vi "RWA_String Section To Anything.vi"(5 "Format String (%#_13g)":string="%#_13g", 6 "Use Supplied":bool, 7 "Read/Write Options":T1={"TS Fmt"="", "Int Fmt"="", "Delimiter"=","}, 8 "Error":errorcluster, 9 "String Section":string, 11 "Type Of Anything":variant) -> (0 "Error Out":errorcluster, 2 "Read Failures Out":string, 3 "Type Of Anything Out":variant, 4 "All Items Found Out":bool)   [LabVIEW 2020]
doc: "Parse the specified String to populate the specified datatype. If string doesn't contain a field defined by datatype, then that field is set based on \"Use Supplied\". If \"Use Supplied\" is true, then the field is left as is, otherwise the field is set to default value.\n\nAuthored by Robert C. Mortensen\nsupport@mooregoodideas.com\nwww.mooregoodideas.com\n\nCopyright (c) 2010, Moore Good Ideas, Inc.\n\nAll rights reserved.\n\nRedistribution and use in source and binary forms, with or without modification, are permitted provided that the following conditions are met:\n\n * Redistributions of source code must retain the above copyright notice, this list of conditions and the following disclaimer.\n * Redistributions in binary form must reproduce the above copyright notice, this list of conditions and the following disclaimer in the documentation and/or other materials provided with the distribution.\n * Neither the name of Moore Good Ideas, Inc. nor the names of its contributors may be used to endorse or promote products derived from this software without specific prior written permission.\n\nTHIS SOFTWARE IS PROVIDED BY THE COPYRIGHT HOLDERS AND CONTRIBUTORS \"AS IS\" AND ANY EXPRESS OR IMPLIED WARRANTIES, INCLUDING, BUT NOT LIMITED TO, THE IMPLIED WARRANTIES OF MERCHANTABILITY AND FITNESS FOR A PARTICULAR PURPOSE ARE DISCLAIMED. IN NO EVENT SHALL THE COPYRIGHT OWNER OR CONTRIBUTORS BE LIABLE FOR ANY DIRECT, INDIRECT, INCIDENTAL, SPECIAL, EXEMPLARY, OR CONSEQUENTIAL DAMAGES (INCLUDING, BUT NOT LIMITED TO, PROCUREMENT OF SUBSTITUTE GOODS OR SERVICES; LOSS OF USE, DATA, OR PROFITS; OR BUSINESS INTERRUPTION) HOWEVER CAUSED AND ON ANY THEORY OF LIABILITY, WHETHER IN CONTRACT, STRICT LIABILITY, OR TORT (INCLUDING NEGLIGENCE OR OTHERWISE) ARISING IN ANY WAY OUT OF THE USE OF THIS SOFTWARE, EVEN IF ADVISED OF THE POSSIBILITY OF SUCH DAMAGE."
uses:
  MGI RWA Options Cluster.ctl
  MGI RWA Convertion Direction Enum.ctl
  <vilib>/Utility/VariantDataType/Type.ctl
  String/MGI Scan From String/MGI Scan From String (CDB).vi
  String/MGI Scan From String/MGI Scan From String (CSG).vi
  String/MGI Scan From String/MGI Scan From String (CXT).vi
  <vilib>/Utility/VariantDataType/VariantType.lvlib
  <vilib>/Utility/Data Type/NI_Data Type.lvlib
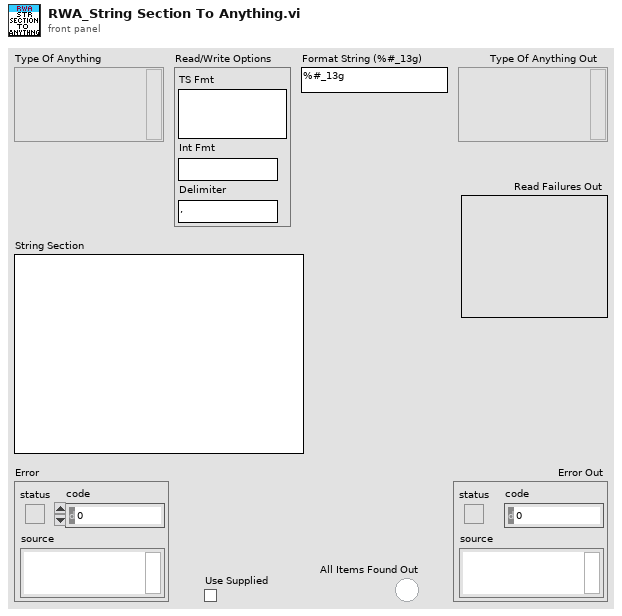
[diagram p1: front panel]
types:
  T1 = typedef "MGI RWA Options Cluster.ctl" = cluster{"TS Fmt":string, "Int Fmt":string, "Delimiter":string}
  T2 = typedef "MGI RWA Convertion Direction Enum.ctl" = enum16{"String->Anything", "Anything->String"}
  T3 = typedef "MGI RWA Tag Lookup Cluster.ctl" = cluster{"StrToSpecifiedText":variant, "Specified Data":variant, "Float Fmt":string, "Major Vers":i32, "Options":T1}
  T4 = typedef "VariantType.lvlib/Type.ctl" = enum8{"Invalid Type", "Void", "I8", "I16", "I32", "I64", "U8", "U16", "U32", "U64", "Single Float", "Double Float", "Extended Float", "Single Complex", "Double Complex", "Extended Complex", "Enum U8", "Enum U16", "Enum U32", "Enum U64", "Single Float With Unit", "Double Float With Unit", "Extended Float With Unit", "Single Complex with Unit", "Double Complex with Unit", "Extended Complex with Unit", "Boolean", "String", "Path", "Picture", "Tag", "Array", "Cluster", "Variant", "LV Variant", "Waveform", "Timestamp", "Digital Waveform", "Digital Data", "ExpressData", "Refnum", "External Data", "VI", "Poly VI", "LabVIEW Class Instance", "Fixed Point"}
  T5 = typedef "NI_Data Type.lvlib/Data Type.ctl" = enum8{"Invalid Type", "Void", "I8", "I16", "I32", "I64", "U8", "U16", "U32", "U64", "Single Float", "Double Float", "Extended Float", "Single Complex", "Double Complex", "Extended Complex", "Enum U8", "Enum U16", "Enum U32", "Enum U64", "Single Float With Unit", "Double Float With Unit", "Extended Float With Unit", "Single Complex with Unit", "Double Complex with Unit", "Extended Complex with Unit", "Boolean", "String", "Path", "Picture", "Tag", "Array", "Cluster", "Variant", "LV Variant", "Waveform", "Timestamp", "Digital Waveform", "Digital Data", "ExpressData", "Refnum", "External Data", "VI", "Poly VI", "LabVIEW Class Instance", "Fixed Point", "Set Collection", "Map Collection"}
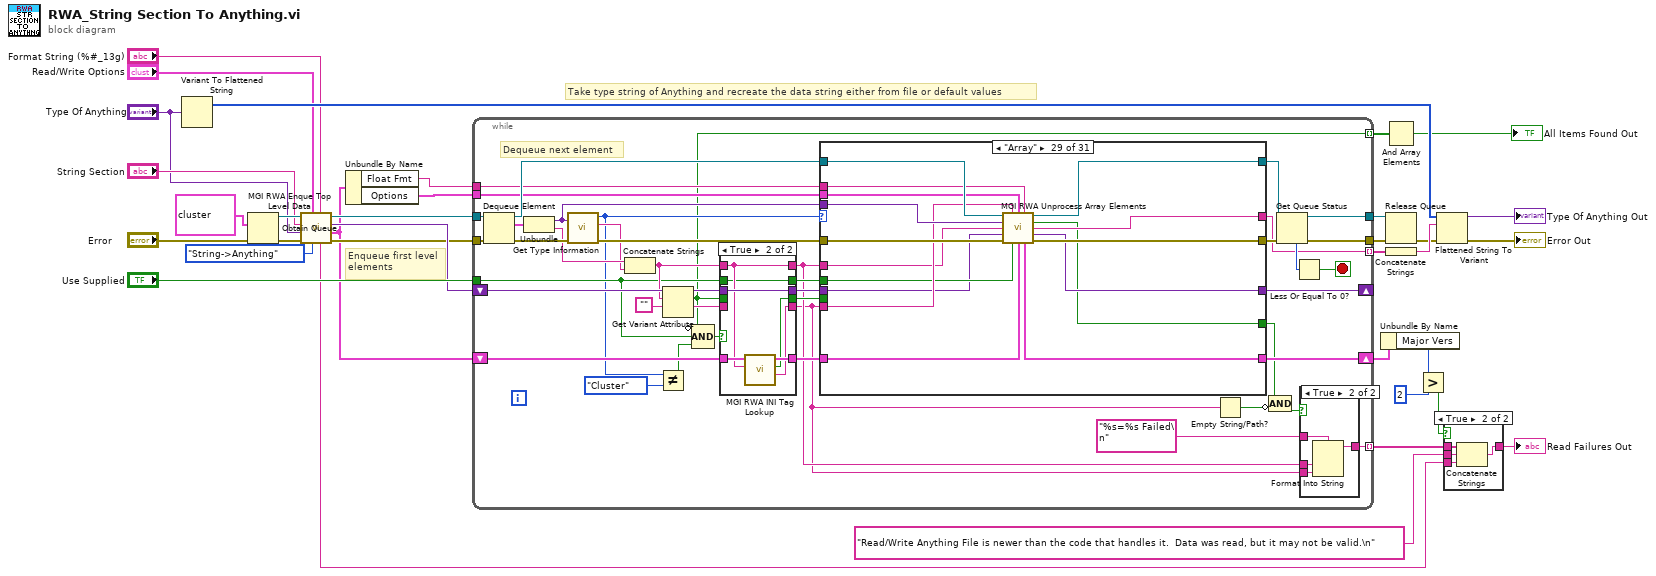
[diagram p0: block diagram]
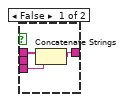
[diagram p2: hidden frame]
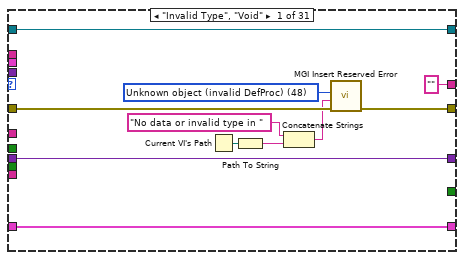
[diagram p5: hidden frame]
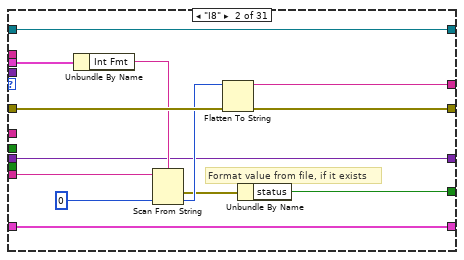
[diagram p6: hidden frame]
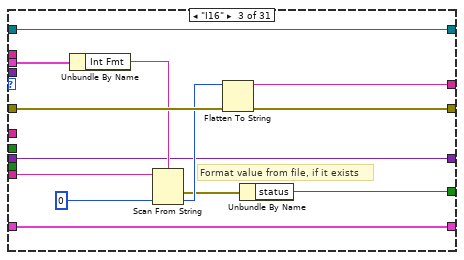
[diagram p7: hidden frame]
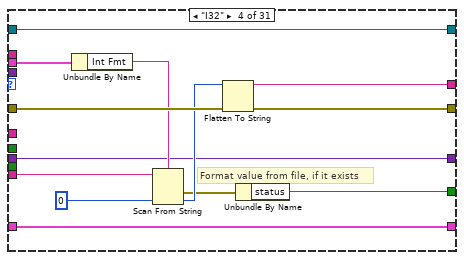
[diagram p8: hidden frame]
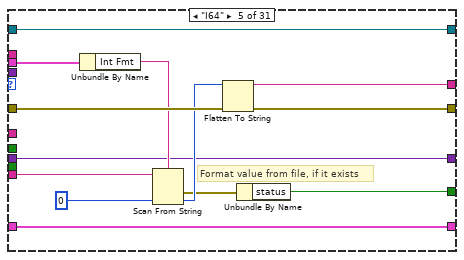
[diagram p9: hidden frame]
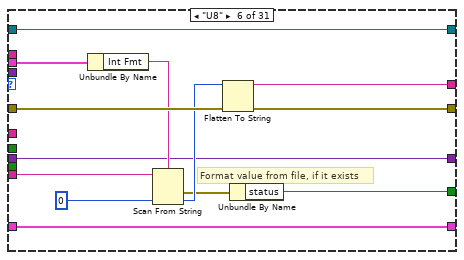
[diagram p10: hidden frame]
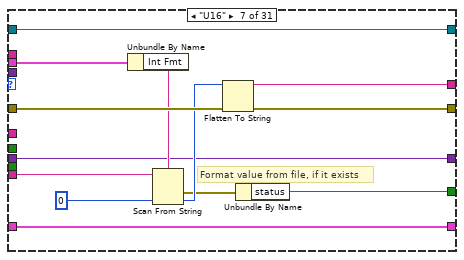
[diagram p11: hidden frame]
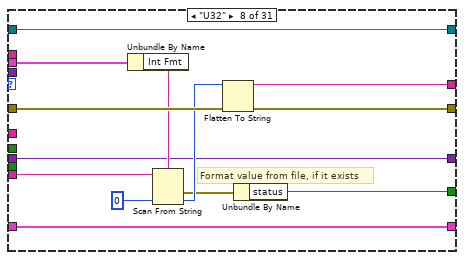
[diagram p12: hidden frame]
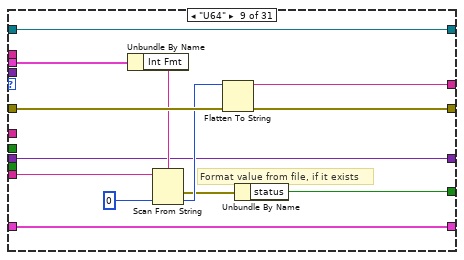
[diagram p13: hidden frame]
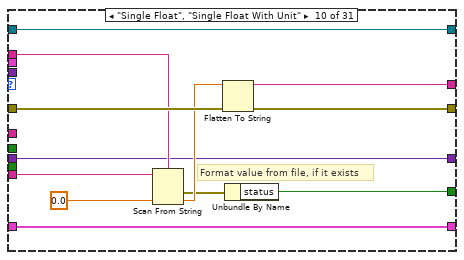
[diagram p14: hidden frame]
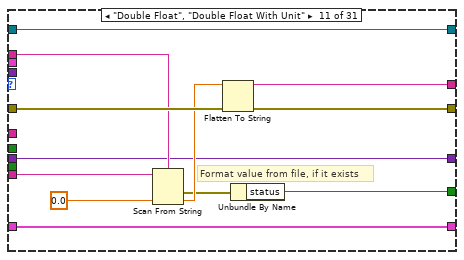
[diagram p15: hidden frame]
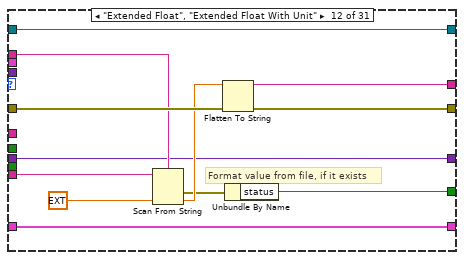
[diagram p16: hidden frame]
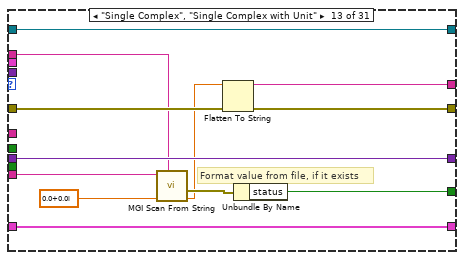
[diagram p17: hidden frame]
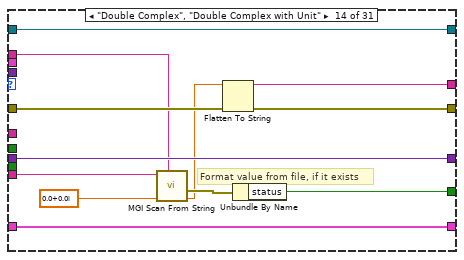
[diagram p18: hidden frame]
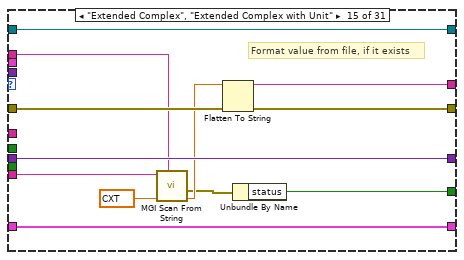
[diagram p19: hidden frame]
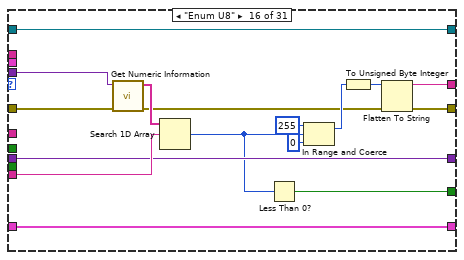
[diagram p20: hidden frame]
diagram:
  # "Enqueue first level\nelements"
  # "Take type string of Anything and recreate the data string either from file or default values"
  n1 = Variant To Flattened String(Variant="Type Of Anything") -> (1:w27:i16[])  [unwired: 1 out]
  n2 = Obtain Queue(element data type=cluster{"Variant":variant, "Name":string} {"Variant"=variant, "Name"=""}, error in (no error)="Error") -> (queue out=w25:refnum<queue>, error out=w19:errorcluster)  [unwired: 3 in, 1 out]
  n3 = call "MGI RWA Enque Top Level Data.vi"("Format String (%#_13g)"="Format String (%#_13g)", "Conversion"=MGI_RWA_Convertion_Direction_Enum."String->Anything", "Read/Write Options"="Read/Write Options", "Error In"=w19, "Anything"="Type Of Anything", "Read String"="String Section", "Data Queue In"=w25) -> ("Error Out"=w22:errorcluster, "Read State"=w17:T3, "Tag to String"=w24:variant, "Data Queue Our"=w23:refnum<queue>, "Warnings"=w3:string)
  n4 = Unbundle By Name(w17) -> ("Float Fmt"=w15:string, "Options"=w13:T1)
  n5 = while {
    tunnel: w22 -> [w76]
    tunnel: [w43] -> w30
    tunnel: [w63] -> w29 mode=indexing
    tunnel: w23 -> [w73]
    tunnel: [w68] -> w32
    tunnel: w13 -> [w45]
    tunnel: w15 -> [w44]
    shift-right: [w50] -> w12
    shift-left: w17 -> [w54]
    shift-right: [w49] -> _
    shift-left: w24 -> [w61]
    tunnel: "Use Supplied" -> [w53]
    tunnel: [w36] -> w8 mode=indexing
    tunnel: [w35] -> w2 mode=indexing
    stop <- w69 stop-if-true
    # "Dequeue next element"
    n6 = Dequeue Element(queue=w73, error in (no error)=w76) -> (queue out=w74:refnum<queue>, element=w67:cluster{"Variant":variant, "Name":string}, error out=w75:errorcluster)  [unwired: 1 in, 1 out]
    n7 = Unbundle(w67) -> ("Variant"=w65:variant, "Name"=w66:string)
    n8 = call <vilib>:"Get Type Information.vi"("error in (no error)"=w75, "variant"=w65) -> ("error out"=w77:errorcluster, "name"=w64:string, "type"=w48:T5)  [unwired: 5 in, 2 out]
    n9 = Concatenate Strings(w66, w64) -> (w58:string)
    n10 = Not Equal?(x=w48, y=Type."Cluster") -> (x != y?=w47:bool)
    n11 = Get Variant Attribute(Variant=w61, name=w58, default value (empty Variant)="") -> (duplicate Variant=w57:variant, found=w35:bool, value=w60:string)  [unwired: 1 in, 1 out]
    n12 = Compound Arithmetic op=AND(invert w35, w53, w47) -> (w59:bool)
    n13 = case shown="True" w59 {
      tunnel: w60 -> [w84 _]
      tunnel: w35 -> [w85 _]
      tunnel: w58 -> [w86 w89]
      tunnel: w57 -> [w87 w93]
      tunnel: [w87 w93] -> w56
      tunnel: [w86 w89] -> w39
      tunnel: [w85 w91] -> w55
      tunnel: [w84 w90] -> w38
      tunnel: w54 -> [w83 w94]
      tunnel: [w83 w92] -> w51
      tunnel: w53 -> [w82 w88]
      tunnel: [w82 w88] -> w52
      frame False {
      }
      frame True {
        n14 = call "MGI RWA INI Tag Lookup.vi"("String"=w89, "State In"=w94) -> ("INI Text"=w90:string, "Text Found?"=w91:bool, "State Out"=w92:T3)  [unwired: 7 in]
      }
    }
    n15 = case shown="\"Array\"" w48 {
      tunnel: [w99 w118 w131 w144 w157 w170 w183 w196 w209 w221 w233 w245 w257 w269 w281 w297 w313 w329 w345 w355 w363 w371 w379 w400 w428 w461 w507 w535 w567 w582 w603] -> w72
      tunnel: w77 -> [w100 w117 w130 w143 w156 w169 w182 w195 w208 w220 w232 w244 w256 w268 w280 w296 w312 w328 w344 w354 w362 w370 w385 w399 w427 w460 w506 w534 w570 w581 w602]
      tunnel: w39 -> [_ _ _ _ _ _ _ _ _ _ _ _ _ _ _ _ _ _ _ _ _ _ w372 _ _ _ _ _ w564 _ _]
      tunnel: ["" ("data string") w116 w129 w142 w155 w168 w181 w194 w207 w219 w231 w243 w255 w267 w279 w295 w311 w327 w343 w353 w361 w369 "" w398 w426 w459 w505 w533 w559 w580 w601] -> w63
      tunnel: w65 -> [_ _ _ _ _ _ _ _ _ _ _ _ _ _ _ w294 w310 w326 w342 _ _ _ w384 _ _ _ _ _ w569 w573 _]
      tunnel: w74 -> [w101 w115 w128 w141 w154 w167 w180 w193 w206 w218 w230 w242 w254 w266 w278 w293 w309 w325 w341 w352 w360 w368 w380 w397 w425 w458 w504 w532 w571 w579 w600]
      tunnel: [w101 w115 w128 w141 w154 w167 w180 w193 w206 w218 w230 w242 w254 w266 w278 w293 w309 w325 w341 w352 w360 w368 w378 w397 w425 w458 w504 w532 w566 w579 w600] -> w71
      tunnel: w56 -> [w96 w110 w123 w136 w149 w162 w175 w188 w202 w213 w225 w237 w253 w265 w277 w285 w301 w318 w333 w347 w358 w365 w374 w395 w422 w451 w501 w529 w563 w574 w597]
      tunnel: w45 -> [_ w108 w121 w134 w147 w160 w173 w186 w199 _ _ _ _ _ _ _ _ _ _ _ _ _ _ _ _ _ _ _ w558 _ _]
      tunnel: w44 -> [_ _ _ _ _ _ _ _ _ w215 w227 w239 w248 w261 w272 _ _ _ _ _ _ _ _ _ _ _ _ _ w557 _ _]
      tunnel: [w96 w110 w123 w136 w149 w162 w175 w188 w202 w213 w225 w237 w253 w265 w277 w285 w301 w318 w333 w347 w358 w365 w374 w395 w422 w451 w501 w529 w560 w574 w597] -> w49
      tunnel: w38 -> [_ w111 w124 w137 w150 w163 w176 w189 w201 w214 w226 w238 w247 w258 w273 w286 w302 w319 w334 w348 w359 w366 _ w396 w424 w452 w502 w530 w568 w577 w598]
      tunnel: w55 -> [_ _ _ _ _ _ _ _ _ _ _ _ _ _ _ _ _ _ _ _ _ _ _ w394 w423 w453 w503 w531 _ w578 w599]
      tunnel: w52 -> [_ _ _ _ _ _ _ _ _ _ _ _ _ _ _ _ _ _ _ _ _ _ _ _ _ _ _ _ w565 _ _]
      tunnel: w51 -> [w95 w109 w122 w135 w148 w161 w174 w187 w200 w212 w224 w236 w252 w264 w276 w284 w300 w317 w332 w346 w357 w364 w373 w393 w421 w450 w500 w528 w562 w576 w596]
      tunnel: [w95 w109 w122 w135 w148 w161 w174 w187 w200 w212 w224 w236 w252 w264 w276 w284 w300 w317 w332 w346 w357 w364 w373 w393 w421 w450 w500 w528 w561 w575 w596] -> w50
      tunnel: [_ w106 w119 w132 w145 w158 w171 w184 w197 w210 w222 w234 w251 w263 w275 w282 w298 w314 w330 _ _ _ _ _ _ w449 _ _ w556 w572 _] -> w42
      frame "Invalid Type", "Void" {
        w97 = u16 48 items=["No error", "Argument error", "Memory is full", "Out of zone", "End of file", "File already open", "Generic file I/O error", "File not found", "File permission error", "Disk is full", "Duplicate path", "Too many files open", "System feature not enabled", "Resource file not found", "Cannot add resource", "Resource not found", "Image not found", "Image memory error", "Pen does not exist", "Config type invalid", "Config token not found", "Config parse error", "Config memory error", "Bad external code format", "Bad external code offset", "External code not present", "Null window", "Destroy window error", "Null menu", "Print aborted", "Bad print record", "Print driver error", "Windows error during printing", "Memory error during printing", "Print dialog error", "Generic print error", "Invalid device refnum", "Device not found", "Device parameter error", "Device unit error", "Cannot open device", "Device call aborted", "Generic error", "Cancelled by user", "Object ID too low", "Object ID too high", "Object not in heap", "Unknown heap", "Unknown object (invalid DefProc)", "Unknown object (DefProc not in table)", "Message out of range", "Invalid (null) method", "Unknown message", "Manager call not supported", "Bad address", "Network operation in progress", "Network operation timed out", "Connection is busy", "Network attribute not supported", "Network error", "Address in use", "System out of memory", "Connection aborted", "Connection refused", "Not connected", "Already connected", "Connection closed", "Initialization error (interapplication manager)", "Bad occurrence", "Wait on unbound occurrence handler", "Occurrence queue overflow", "Datalog type conflict", "Unused", "Unrecognized type (interapplication manager)", "Memory corrupt", "Failed to make temporary DLL", "Old CIN version", "Drag socket not found", "Failed to load drop-object", "Failed to register OLE object", "Failed to release OLE object", "Format specifier type mismatch", "Unknown format specifier", "Too few format specifiers", "Too many format specifiers", "Scan failed", "Newer CIN version", "OLE Convert", "Runtime menu error", "Password tampered", "Unknown error code"] ("Reserved Error Code")
        n16 = Current VI's Path() -> (path=w103:path)
        n17 = Path To String(path=w103) -> (string=w102:string)
        n18 = Concatenate Strings("No data or invalid type in " ("string"), w102) -> (w98:string)
        n19 = call "MGI Insert Reserved Error.vi"("Error In"=w100, "Error Description"=w98, "Reserved Error Code (Generic error)"=w97) -> ("Error Out"=w99:errorcluster)  [unwired: 8 in]
      }
      frame "I8" {
        # "Format value from file, if it exists"
        n20 = Unbundle By Name(w108) -> ("Int Fmt"=w113:string)
        n21 = Scan From String(format string=w113, input string=w111, default 1=i8 0 ("default (0 I32)")) -> (error out=w107:errorcluster, output 1=w112:i8)  [unwired: 2 in, 2 out]
        n22 = Flatten To String(anything=w112, error in (no error)=w117) -> (data string=w116:string, error out=w118:errorcluster)  [unwired: 2 in, 1 out]
        n23 = Unbundle By Name(w107) -> ("status"=w106:bool)
      }
      frame "I16" {
        # "Format value from file, if it exists"
        n24 = Unbundle By Name(w121) -> ("Int Fmt"=w126:string)
        n25 = Scan From String(format string=w126, input string=w124, default 1=i16 0 ("default (0 I32)")) -> (error out=w120:errorcluster, output 1=w125:i16)  [unwired: 2 in, 2 out]
        n26 = Flatten To String(anything=w125, error in (no error)=w130) -> (data string=w129:string, error out=w131:errorcluster)  [unwired: 2 in, 1 out]
        n27 = Unbundle By Name(w120) -> ("status"=w119:bool)
      }
      frame "I32" {
        # "Format value from file, if it exists"
        n28 = Unbundle By Name(w134) -> ("Int Fmt"=w139:string)
        n29 = Scan From String(format string=w139, input string=w137, default 1=0 ("default (0 I32)")) -> (error out=w133:errorcluster, output 1=w138:i32)  [unwired: 2 in, 2 out]
        n30 = Flatten To String(anything=w138, error in (no error)=w143) -> (data string=w142:string, error out=w144:errorcluster)  [unwired: 2 in, 1 out]
        n31 = Unbundle By Name(w133) -> ("status"=w132:bool)
      }
      frame "I64" {
        # "Format value from file, if it exists"
        n32 = Unbundle By Name(w147) -> ("Int Fmt"=w152:string)
        n33 = Scan From String(format string=w152, input string=w150, default 1=i64 0 ("default (0 I32)")) -> (error out=w146:errorcluster, output 1=w151:i64)  [unwired: 2 in, 2 out]
        n34 = Flatten To String(anything=w151, error in (no error)=w156) -> (data string=w155:string, error out=w157:errorcluster)  [unwired: 2 in, 1 out]
        n35 = Unbundle By Name(w146) -> ("status"=w145:bool)
      }
      frame "U8" {
        # "Format value from file, if it exists"
        n36 = Unbundle By Name(w160) -> ("Int Fmt"=w165:string)
        n37 = Scan From String(format string=w165, input string=w163, default 1=u8 0 ("default (0 I32)")) -> (error out=w159:errorcluster, output 1=w164:u8)  [unwired: 2 in, 2 out]
        n38 = Flatten To String(anything=w164, error in (no error)=w169) -> (data string=w168:string, error out=w170:errorcluster)  [unwired: 2 in, 1 out]
        n39 = Unbundle By Name(w159) -> ("status"=w158:bool)
      }
      frame "U16" {
        # "Format value from file, if it exists"
        n40 = Unbundle By Name(w173) -> ("Int Fmt"=w178:string)
        n41 = Scan From String(format string=w178, input string=w176, default 1=u16 0 ("default (0 I32)")) -> (error out=w172:errorcluster, output 1=w177:u16)  [unwired: 2 in, 2 out]
        n42 = Flatten To String(anything=w177, error in (no error)=w182) -> (data string=w181:string, error out=w183:errorcluster)  [unwired: 2 in, 1 out]
        n43 = Unbundle By Name(w172) -> ("status"=w171:bool)
      }
      frame "U32" {
        # "Format value from file, if it exists"
        n44 = Unbundle By Name(w186) -> ("Int Fmt"=w191:string)
        n45 = Scan From String(format string=w191, input string=w189, default 1=u32 0 ("default (0 I32)")) -> (error out=w185:errorcluster, output 1=w190:u32)  [unwired: 2 in, 2 out]
        n46 = Flatten To String(anything=w190, error in (no error)=w195) -> (data string=w194:string, error out=w196:errorcluster)  [unwired: 2 in, 1 out]
        n47 = Unbundle By Name(w185) -> ("status"=w184:bool)
      }
      frame "U64" {
        # "Format value from file, if it exists"
        n48 = Unbundle By Name(w199) -> ("Int Fmt"=w204:string)
        n49 = Scan From String(format string=w204, input string=w201, default 1=u64 0 ("default (0 I32)")) -> (error out=w198:errorcluster, output 1=w203:u64)  [unwired: 2 in, 2 out]
        n50 = Flatten To String(anything=w203, error in (no error)=w208) -> (data string=w207:string, error out=w209:errorcluster)  [unwired: 2 in, 1 out]
        n51 = Unbundle By Name(w198) -> ("status"=w197:bool)
      }
      frame "Single Float", "Single Float With Unit" {
        # "Format value from file, if it exists"
        n52 = Scan From String(format string=w215, input string=w214, default 1=sgl 0.0 ("default (0 I32)")) -> (error out=w211:errorcluster, output 1=w216:sgl)  [unwired: 2 in, 2 out]
        n53 = Flatten To String(anything=w216, error in (no error)=w220) -> (data string=w219:string, error out=w221:errorcluster)  [unwired: 2 in, 1 out]
        n54 = Unbundle By Name(w211) -> ("status"=w210:bool)
      }
      frame "Double Float", "Double Float With Unit" {
        # "Format value from file, if it exists"
        n55 = Scan From String(format string=w227, input string=w226, default 1=0.0 ("default (0 I32)")) -> (error out=w223:errorcluster, output 1=w228:dbl)  [unwired: 2 in, 2 out]
        n56 = Flatten To String(anything=w228, error in (no error)=w232) -> (data string=w231:string, error out=w233:errorcluster)  [unwired: 2 in, 1 out]
        n57 = Unbundle By Name(w223) -> ("status"=w222:bool)
      }
      frame "Extended Float", "Extended Float With Unit" {
        # "Format value from file, if it exists"
        n58 = Scan From String(format string=w239, input string=w238, default 1=ext 0.0 ("default (0 I32)")) -> (error out=w235:errorcluster, output 1=w240:ext)  [unwired: 2 in, 2 out]
        n59 = Flatten To String(anything=w240, error in (no error)=w244) -> (data string=w243:string, error out=w245:errorcluster)  [unwired: 2 in, 1 out]
        n60 = Unbundle By Name(w235) -> ("status"=w234:bool)
      }
      frame "Single Complex", "Single Complex with Unit" {
        # "Format value from file, if it exists"
        n61 = call-poly "MGI Scan From String.vi"("format string"=w248, "Default CSG[]"=csg 0.0+0.0i ("default (0 I32)"), "String In"=w247) -> ("CSG[] Out"=w249:csg, "error out"=w250:errorcluster)  [unwired: 5 in, 2 out]
        n62 = Flatten To String(anything=w249, error in (no error)=w256) -> (data string=w255:string, error out=w257:errorcluster)  [unwired: 2 in, 1 out]
        n63 = Unbundle By Name(w250) -> ("status"=w251:bool)
      }
      frame "Double Complex", "Double Complex with Unit" {
        # "Format value from file, if it exists"
        n64 = call-poly "MGI Scan From String.vi"("format string"=w261, "Default CXT[]"=cdb 0.0+0.0i ("default (0 I32)"), "String In"=w258) -> ("CXT[] Out"=w259:cdb, "error out"=w260:errorcluster)  [unwired: 5 in, 2 out]
        n65 = Flatten To String(anything=w259, error in (no error)=w268) -> (data string=w267:string, error out=w269:errorcluster)  [unwired: 2 in, 1 out]
        n66 = Unbundle By Name(w260) -> ("status"=w263:bool)
      }
      frame "Extended Complex", "Extended Complex with Unit" {
        # "Format value from file, if it exists"
        n67 = call-poly "MGI Scan From String.vi"("format string"=w272, "Default CXT[]"=cxt 0.0+0.0i ("default (0 I32)"), "String In"=w273) -> ("CXT[] Out"=w271:cxt, "error out"=w270:errorcluster)  [unwired: 5 in, 2 out]
        n68 = Flatten To String(anything=w271, error in (no error)=w280) -> (data string=w279:string, error out=w281:errorcluster)  [unwired: 2 in, 1 out]
        n69 = Unbundle By Name(w270) -> ("status"=w275:bool)
      }
      frame "Enum U8" {
        n70 = call <vilib>:"Get Numeric Information.vi"("error in (no error)"=w296, "variant"=w294) -> ("error out"=w287:errorcluster, "enum names"=w292:string[])  [unwired: 6 in, 2 out]
        n71 = Search 1D Array(1D array=w292, element=w286) -> (index of element=w283:i32)  [unwired: 1 in]
        n72 = Less Than 0?(x=w283) -> (x < 0?=w282:bool)
        n73 = In Range and Coerce(upper limit=255, x=w283, lower limit=0) -> (coerced(x)=w290:i32)  [unwired: 1 out]
        n74 = To Unsigned Byte Integer(number=w290) -> (unsigned 8bit integer=w291:u8)
        n75 = Flatten To String(anything=w291, error in (no error)=w287) -> (data string=w295:string, error out=w297:errorcluster)  [unwired: 2 in, 1 out]
      }
      frame "Enum U16" {
        n76 = call <vilib>:"Get Numeric Information.vi"("error in (no error)"=w312, "variant"=w310) -> ("error out"=w306:errorcluster, "enum names"=w308:string[])  [unwired: 6 in, 2 out]
        n77 = Search 1D Array(1D array=w308, element=w302) -> (index of element=w299:i32)  [unwired: 1 in]
        n78 = In Range and Coerce(upper limit=65535, x=w299, lower limit=0) -> (coerced(x)=w304:i32)  [unwired: 1 out]
        n79 = Less Than 0?(x=w299) -> (x < 0?=w298:bool)
        n80 = To Unsigned Word Integer(number=w304) -> (unsigned 16bit integer=w303:u16)
        n81 = Flatten To String(anything=w303, error in (no error)=w306) -> (data string=w311:string, error out=w313:errorcluster)  [unwired: 2 in, 1 out]
      }
      frame "Enum U32" {
        n82 = call <vilib>:"Get Numeric Information.vi"("error in (no error)"=w328, "variant"=w326) -> ("error out"=w322:errorcluster, "enum names"=w324:string[])  [unwired: 6 in, 2 out]
        n83 = Search 1D Array(1D array=w324, element=w319) -> (index of element=w315:i32)  [unwired: 1 in]
        n84 = Less Than 0?(x=w315) -> (x < 0?=w314:bool)
        n85 = In Range and Coerce(upper limit=2147483647, x=w315, lower limit=0) -> (coerced(x)=w321:i32)  [unwired: 1 out]
        n86 = To Unsigned Long Integer(number=w321) -> (unsigned 32bit integer=w320:u32)
        n87 = Flatten To String(anything=w320, error in (no error)=w322) -> (data string=w327:string, error out=w329:errorcluster)  [unwired: 2 in, 1 out]
      }
      frame "Enum U64" {
        n88 = call <vilib>:"Get Numeric Information.vi"("error in (no error)"=w344, "variant"=w342) -> ("error out"=w338:errorcluster, "enum names"=w340:string[])  [unwired: 6 in, 2 out]
        n89 = Search 1D Array(1D array=w340, element=w334) -> (index of element=w331:i32)  [unwired: 1 in]
        n90 = Less Than 0?(x=w331) -> (x < 0?=w330:bool)
        n91 = In Range and Coerce(upper limit=2147483647, x=w331, lower limit=0) -> (coerced(x)=w335:i32)  [unwired: 1 out]
        n92 = To Unsigned Quad Integer(1:w335) -> (0:w336:u64)
        n93 = Flatten To String(anything=w336, error in (no error)=w338) -> (data string=w343:string, error out=w345:errorcluster)  [unwired: 2 in, 1 out]
      }
      frame "Boolean" {
        n94 = call <vilib>:"Trim Whitespace.vi"("string"=w348) -> ("trimmed string"=w350:string)  [unwired: 1 in]
        n95 = To Upper Case(1:w350) -> (0:w349:string)
        n96 = case shown="Default" w349 {
          tunnel: [_ TRUE] -> w351
          frame Default {
          }
          frame "1", "ON", "TRUE", "YES" {
          }
        }
        n97 = Flatten To String(anything=w351, error in (no error)=w354) -> (data string=w353:string, error out=w355:errorcluster)  [unwired: 2 in, 1 out]
      }
      frame "String" {
        n98 = Flatten To String(anything=w359, error in (no error)=w362) -> (data string=w361:string, error out=w363:errorcluster)  [unwired: 2 in, 1 out]
      }
      frame "Path" {
        n99 = String To Path(string=w366) -> (path=w367:path)
        n100 = Flatten To String(anything=w367, error in (no error)=w370) -> (data string=w369:string, error out=w371:errorcluster)  [unwired: 2 in, 1 out]
      }
      frame "Cluster" {
        # "Enqueue cluster elements"
        n101 = call <vilib>:"Get Cluster Information.vi"("error in (no error)"=w385, "variant"=w384) -> ("error out"=w381:errorcluster, "cluster elements"=w383:variant[])  [unwired: 8 in]
        n102 = Concatenate Strings(w372, "." ("string")) -> (w375:string)
        n103 = Reverse 1D Array(array=w383) -> (reversed array=w382:variant[])
        n104 = for {
          tunnel: w380 -> [w392]
          tunnel: w381 -> [w391]
          tunnel: [w390] -> w379
          tunnel: [w389] -> w378
          tunnel: w382 -> [w388] mode=indexing
          tunnel: w375 -> [w386]
          n105 = Bundle("Variant"=w388, w386) -> (w387:cluster{"Variant":variant, string})  [unwired: 1 in]
          n106 = Enqueue Element At Opposite End(queue=w392, element=w387, error in (no error)=w391) -> (queue out=w389:refnum<queue>, error out=w390:errorcluster)  [unwired: 1 in, 1 out]
        }
      }
      frame "Variant", "LV Variant" {
        n107 = case shown="True" w394 {
          tunnel: w396 -> [w401 _]
          tunnel: [w409 w418] -> w400
          tunnel: w399 -> [w409 w419]
          tunnel: [w407 w420] -> w398
          frame True {
            n108 = String Subset(string=w401, offset (0)=2) -> (substring=w406:string)  [unwired: 1 in]
            n109 = String Length(string=w406) -> (length=w404:i32)
            n110 = Multiply(x=0.5, y=w404) -> (x*y=w403:dbl)
            n111 = for {
              N: w403 -> [_]
              tunnel: w406 -> [w413]
              tunnel: [w415] -> w405 mode=indexing
              i -> [w412]
              w411 = 2 ("length (rest)")
              n112 = Multiply(x=w412, y=w411) -> (x*y=w410:i32)
              n113 = String Subset(string=w413, offset (0)=w410, length (rest)=w411) -> (substring=w414:string)
              n114 = Hexadecimal String To Number(string=w414, default (0uL)=u8 0 ("default (0 U32)")) -> (number=w415:u8)  [unwired: 1 in, 1 out]
            }
            n115 = Byte Array To String(unsigned byte array=w405) -> (string=w407:string)
          }
          frame False {
            w417 = variant  # Variant
            n116 = Flatten To String(anything=w417, error in (no error)=w419) -> (data string=w420:string, error out=w418:errorcluster)  [unwired: 2 in, 1 out]
          }
        }
      }
      frame "Waveform" {
        n117 = case shown="True" w423 {
          tunnel: w424 -> [w429 _]
          tunnel: [w437 w447] -> w428
          tunnel: w427 -> [w437 w446]
          tunnel: [w435 w448] -> w426
          frame True {
            n118 = String Subset(string=w429, offset (0)=2) -> (substring=w434:string)  [unwired: 1 in]
            n119 = String Length(string=w434) -> (length=w432:i32)
            n120 = Multiply(x=0.5, y=w432) -> (x*y=w431:dbl)
            n121 = for {
              N: w431 -> [_]
              tunnel: w434 -> [w441]
              tunnel: [w443] -> w433 mode=indexing
              i -> [w440]
              w439 = 2 ("length (rest)")
              n122 = Multiply(x=w440, y=w439) -> (x*y=w438:i32)
              n123 = String Subset(string=w441, offset (0)=w438, length (rest)=w439) -> (substring=w442:string)
              n124 = Hexadecimal String To Number(string=w442, default (0uL)=u8 0 ("default (0 U32)")) -> (number=w443:u8)  [unwired: 1 in, 1 out]
            }
            n125 = Byte Array To String(unsigned byte array=w433) -> (string=w435:string)
          }
          frame False {
            n126 = Flatten To String(anything=waveform(dbl) {"t0"=timestamp(0 s since 1904-01-01), "dt"=0.0, "Y"=[]} ("Waveform 2"), error in (no error)=w446) -> (data string=w448:string, error out=w447:errorcluster)  [unwired: 2 in, 1 out]
          }
        }
      }
      frame "Timestamp" {
        n127 = Unbundle By Name(w450) -> ("Options.TS Fmt"=w457:string)
        n128 = Match First String(2:string[] ["0x"] ("string array"), 3:w452) -> (0:w455:i32, 1:w454:string)
        n129 = case shown="True" w453 {
          tunnel: [w464 w498] -> w461
          tunnel: w460 -> [w465 w497]
          tunnel: [w468 w499] -> w459
          tunnel: w457 -> [w467 _]
          tunnel: w455 -> [w463 _]
          tunnel: w454 -> [w466 _]
          tunnel: [w462 _] -> w449
          frame True {
            n130 = case shown="0.." w463 {
              tunnel: [w471 w493] -> w468
              tunnel: w467 -> [_ w489]
              tunnel: w466 -> [w473 w492]
              tunnel: w465 -> [w472 w491]
              tunnel: [w472 w490] -> w464
              tunnel: [FALSE ("status") w484] -> w462
              frame 0.. {
                n131 = String Length(string=w473) -> (length=w474:i32)
                n132 = Quotient & Remainder(x=w474, y=2) -> (floor(x/y)=w476:i32)  [unwired: 1 out]
                n133 = for {
                  N: w476 -> [_]
                  tunnel: w473 -> [w480]
                  tunnel: [w482] -> w470 mode=indexing
                  i -> [w479]
                  w478 = 2 ("length (rest)")
                  n134 = Multiply(x=w479, y=w478) -> (x*y=w477:i32)
                  n135 = String Subset(string=w480, offset (0)=w477, length (rest)=w478) -> (substring=w481:string)
                  n136 = Hexadecimal String To Number(string=w481, default (0uL)=u8 0 ("default (0 U32)")) -> (number=w482:u8)  [unwired: 1 in, 1 out]
                }
                n137 = Byte Array To String(unsigned byte array=w470) -> (string=w471:string)
              }
              frame ..-1 {
                n138 = Concatenate Strings("%<" ("string"), w489, ">T" ("string")) -> (w488:string)
                n139 = Scan From String(format string=w488, input string=w492, default 1=timestamp(0 s since 1904-01-01)) -> (error out=w485:errorcluster, output 1=w494:timestamp)  [unwired: 2 in, 2 out]
                n140 = Unbundle By Name(w485) -> ("status"=w484:bool)
                n141 = Flatten To String(anything=w494, error in (no error)=w491) -> (data string=w493:string, error out=w490:errorcluster)  [unwired: 2 in, 1 out]
              }
            }
          }
          frame False {
            n142 = Flatten To String(anything=timestamp(0 s since 1904-01-01), error in (no error)=w497) -> (data string=w499:string, error out=w498:errorcluster)  [unwired: 2 in, 1 out]
          }
        }
      }
      frame "Digital Waveform" {
        n143 = case shown="True" w503 {
          tunnel: w502 -> [w508 _]
          tunnel: [w516 w526] -> w507
          tunnel: w506 -> [w516 w525]
          tunnel: [w514 w527] -> w505
          frame True {
            n144 = String Subset(string=w508, offset (0)=2) -> (substring=w513:string)  [unwired: 1 in]
            n145 = String Length(string=w513) -> (length=w511:i32)
            n146 = Multiply(x=0.5, y=w511) -> (x*y=w510:dbl)
            n147 = for {
              N: w510 -> [_]
              tunnel: w513 -> [w520]
              tunnel: [w522] -> w512 mode=indexing
              i -> [w519]
              w518 = 2 ("length (rest)")
              n148 = Multiply(x=w519, y=w518) -> (x*y=w517:i32)
              n149 = String Subset(string=w520, offset (0)=w517, length (rest)=w518) -> (substring=w521:string)
              n150 = Hexadecimal String To Number(string=w521, default (0uL)=u8 0 ("default (0 U32)")) -> (number=w522:u8)  [unwired: 1 in, 1 out]
            }
            n151 = Byte Array To String(unsigned byte array=w512) -> (string=w514:string)
          }
          frame False {
            n152 = call <vilib>:"DWDT Empty Digital.vi"() -> ("digital waveform out"=w524:digitalwaveform)  [unwired: 5 in]
            n153 = Flatten To String(anything=w524, error in (no error)=w525) -> (data string=w527:string, error out=w526:errorcluster)  [unwired: 2 in, 1 out]
          }
        }
      }
      frame "Digital Data" {
        n154 = case shown="True" w531 {
          tunnel: w530 -> [w536 _]
          tunnel: [w544 w554] -> w535
          tunnel: w534 -> [w544 w553]
          tunnel: [w542 w555] -> w533
          frame True {
            n155 = String Subset(string=w536, offset (0)=2) -> (substring=w541:string)  [unwired: 1 in]
            n156 = String Length(string=w541) -> (length=w539:i32)
            n157 = Multiply(x=0.5, y=w539) -> (x*y=w538:dbl)
            n158 = for {
              N: w538 -> [_]
              tunnel: w541 -> [w548]
              tunnel: [w550] -> w540 mode=indexing
              i -> [w547]
              w546 = 2 ("length (rest)")
              n159 = Multiply(x=w547, y=w546) -> (x*y=w545:i32)
              n160 = String Subset(string=w548, offset (0)=w545, length (rest)=w546) -> (substring=w549:string)
              n161 = Hexadecimal String To Number(string=w549, default (0uL)=u8 0 ("default (0 U32)")) -> (number=w550:u8)  [unwired: 1 in, 1 out]
            }
            n162 = Byte Array To String(unsigned byte array=w540) -> (string=w542:string)
          }
          frame False {
            n163 = call <vilib>:"DTbl Empty Digital.vi"() -> ("digital data"=w552:digitaldata)  [unwired: 5 in]
            n164 = Flatten To String(anything=w552, error in (no error)=w553) -> (data string=w555:string, error out=w554:errorcluster)  [unwired: 2 in, 1 out]
          }
        }
      }
      frame "Array" {
        n165 = call "MGI RWA Unprocess Array Elements.vi"("Queue In"=w571, "Value"=w568, "Read/Write Options"=w558, "Format String (%#_13g)"=w557, "Array Variant"=w569, "Name In"=w564, "Str to INI in"=w563, "Error In"=w570, "Use Specified?"=w565, "State In"=w562) -> ("Queue Out"=w566:refnum<queue>, "Scan Failed?"=w556:bool, "Data Out"=w559:string, "Str to INI out"=w560:variant, "State Out"=w561:T3, "Error Out"=w567:errorcluster)
      }
      frame "Tag", "Refnum" {
        n166 = case shown="True" w578 {
          tunnel: w577 -> [w588 _]
          tunnel: [w585 w593] -> w582
          tunnel: w581 -> [w585 w594]
          tunnel: [w590 w595] -> w580
          tunnel: w576 -> [w589 w591]
          tunnel: [w589 w591] -> w575
          tunnel: w574 -> [_ _]
          tunnel: w573 -> [w586 _]
          tunnel: [w583 _] -> w572
          frame True {
            n167 = call "MGI RWA Handle Tag or Refnum.vi"("Read State In"=w589, "Conversion"=MGI_RWA_Convertion_Direction_Enum."String->Anything", "Anything"=w586, "Read String"=w588) -> ("Error Out"=w584:errorcluster, "String"=w590:string)  [unwired: 6 in]
            n168 = Unbundle By Name(w584) -> ("status"=w583:bool)
          }
          frame False {
            n169 = Flatten To String(anything="", error in (no error)=w594) -> (data string=w595:string, error out=w593:errorcluster)  [unwired: 2 in, 1 out]
          }
        }
      }
      frame Default {
        n170 = case shown="True" w599 {
          tunnel: w598 -> [w604 _]
          tunnel: [w612 w621] -> w603
          tunnel: w602 -> [w612 w622]
          tunnel: [w610 w623] -> w601
          frame True {
            n171 = String Subset(string=w604, offset (0)=2) -> (substring=w609:string)  [unwired: 1 in]
            n172 = String Length(string=w609) -> (length=w607:i32)
            n173 = Multiply(x=0.5, y=w607) -> (x*y=w605:dbl)
            n174 = for {
              N: w605 -> [_]
              tunnel: w609 -> [w616]
              tunnel: [w618] -> w608 mode=indexing
              i -> [w615]
              w614 = 2 ("length (rest)")
              n175 = Multiply(x=w615, y=w614) -> (x*y=w613:i32)
              n176 = String Subset(string=w616, offset (0)=w613, length (rest)=w614) -> (substring=w617:string)
              n177 = Hexadecimal String To Number(string=w617, default (0uL)=u8 0 ("default (0 U32)")) -> (number=w618:u8)  [unwired: 1 in, 1 out]
            }
            n178 = Byte Array To String(unsigned byte array=w608) -> (string=w610:string)
          }
          frame False {
            n179 = Flatten To String(anything="", error in (no error)=w622) -> (data string=w623:string, error out=w621:errorcluster)  [unwired: 2 in, 1 out]
          }
        }
      }
    }
    n180 = Empty String/Path?(string/path=w38) -> (empty?=w41:bool)
    n181 = Compound Arithmetic op=AND(w42, invert w41) -> (w40:bool)
    n182 = Get Queue Status(queue=w71, error in (no error)=w72) -> (queue out=w68:refnum<queue>, error out=w43:errorcluster, # elements in queue=w70:i32)  [unwired: 1 in, 5 out]
    n183 = Less Or Equal To 0?(x=w70) -> (x <= 0?=w69:bool)
    n184 = case shown="True" w40 {
      tunnel: w39 -> [_ w81]
      tunnel: w38 -> [_ w80]
      tunnel: "%s=%s Failed\n" ("Error Description") -> [_ w79]
      tunnel: [_ w78] -> w36
      frame False {
      }
      frame True {
        n185 = Format Into String(format string=w79, w81, w80) -> (resulting string=w78:string)  [unwired: 2 in, 1 out]
      }
    }
  }
  n186 = Unbundle By Name(w12) -> ("Major Vers"=w10:i32)
  n187 = And Array Elements(Boolean array=w2) -> (logical AND=→"All Items Found Out":bool)
  n188 = Release Queue(queue=w32, error in (no error)=w30) -> (error out=w31:errorcluster)  [unwired: 1 in, 2 out]
  n189 = Concatenate Strings(w29) -> (w34:string)
  n190 = Greater?(x=w10, y=2) -> (0:w7:bool)
  n191 = Flattened String To Variant(4:w31, 6:w34, 7:w27) -> (0:→"Error Out":errorcluster, 3:→"Type Of Anything Out":variant)
  n192 = case shown="True" w7 {
    tunnel: w8 -> [w626 w630]
    tunnel: "Read/Write Anything File is newer than the code that handles it.  Data was read, but it may not be valid.\n" ("Error Description") -> [_ w629]
    tunnel: [w625 w628] -> w5
    tunnel: w3 -> [w624 w627]
    frame False {
      n193 = Concatenate Strings(w626, w624) -> (w625:string)
    }
    frame True {
      n194 = Concatenate Strings(w630, w629, w627) -> (w628:string)
    }
  }
  "Read Failures Out" <- w5
